vi "Instrument.Cryostat Class Paths.vi"(7 "instrument":T1) -> (0 "Level Path":path, 1 "Rotator Path":path, 2 "Magnet Path":path, 3 "Temperature Path":path)   [LabVIEW 2016, in "Control Experiment.lvclass"]
uses:
  Control Experiment.lvclass
  Typedefs/Instrument--enum.ctl
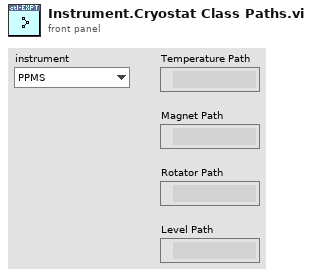
[diagram p1: front panel]
types:
  T1 = typedef "Control Experiment.lvclass/Instrument--enum.ctl" = enum16{"PPMS", "PPMS2", "MFP3D", "CYPHER", "THz1", "THz2", "MNK", "CF900", "JEOL", "AGILENT"}
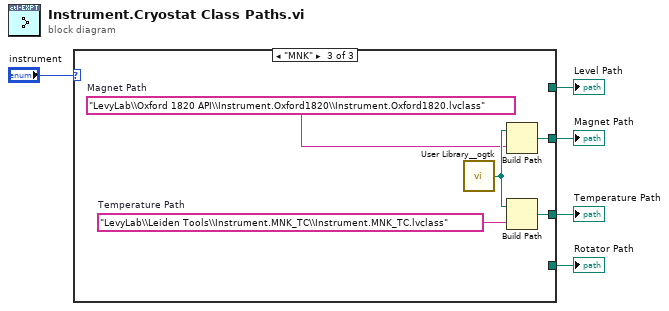
[diagram p0: block diagram]
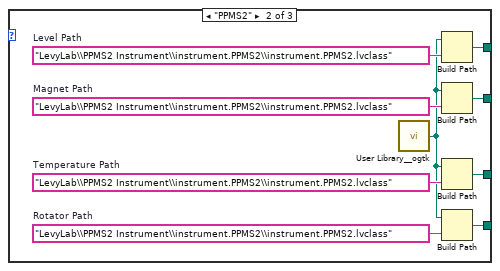
[diagram p3: hidden frame]
diagram:
  n1 = case shown="\"MNK\"" "instrument" {
    tunnel: [_ w13 w18] -> w2
    tunnel: [_ w11 w17] -> w1
    tunnel: [_ w9 _] -> w4
    tunnel: [_ w7 _] -> w3
    frame Default {
    }
    frame "PPMS2" {
      w8 = "LevyLab\\PPMS2 Instrument\\instrument.PPMS2\\instrument.PPMS2.lvclass"  # Level Path
      w10 = "LevyLab\\PPMS2 Instrument\\instrument.PPMS2\\instrument.PPMS2.lvclass"  # Rotator Path
      w12 = "LevyLab\\PPMS2 Instrument\\instrument.PPMS2\\instrument.PPMS2.lvclass"  # Magnet Path
      w14 = "LevyLab\\PPMS2 Instrument\\instrument.PPMS2\\instrument.PPMS2.lvclass"  # Temperature Path
      n2 = call <userlib>:"User Library__ogtk.vi"() -> ("User Library (+ Relative)"=w6:path)  [unwired: 1 in]
      n3 = Build Path(base path=w6, name or relative path=w8) -> (appended path=w7:path)
      n4 = Build Path(base path=w6, name or relative path=w12) -> (appended path=w11:path)
      n5 = Build Path(base path=w6, name or relative path=w14) -> (appended path=w13:path)
      n6 = Build Path(base path=w6, name or relative path=w10) -> (appended path=w9:path)
    }
    frame "MNK" {
      w15 = "LevyLab\\Oxford 1820 API\\Instrument.Oxford1820\\Instrument.Oxford1820.lvclass"  # Magnet Path
      w19 = "LevyLab\\Leiden Tools\\Instrument.MNK_TC\\Instrument.MNK_TC.lvclass"  # Temperature Path
      n7 = call <userlib>:"User Library__ogtk.vi"() -> ("User Library (+ Relative)"=w16:path)  [unwired: 1 in]
      n8 = Build Path(base path=w16, name or relative path=w15) -> (appended path=w17:path)
      n9 = Build Path(base path=w16, name or relative path=w19) -> (appended path=w18:path)
    }
  }
  "Magnet Path" <- w1
  "Temperature Path" <- w2
  "Rotator Path" <- w4
  "Level Path" <- w3
